vi "myArray.vi"() -> ()   [LabVIEW 2014]
panel:
  in  "n":i32
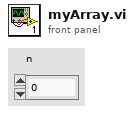
[diagram p1: front panel]
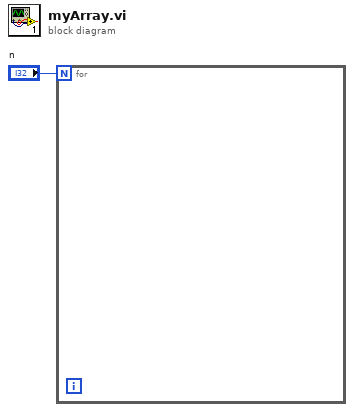
[diagram p0: block diagram]
diagram:
  n1 = for {
    N: "n" -> [_]
  }
